vi "User Authentication Schemes Length.vi"(8 "Error In":errorcluster, 10 "Username":string, 11 "Session In":refnum<class "Session.lvclass">) -> (0 "Error Out":errorcluster, 2 "Length":i32, 3 "Sesssion Out":refnum<class "Session.lvclass">)   [LabVIEW 2017, in "Toolkit.lvlib" / "Session.lvclass"]
uses:
  Session.lvclass
  Session.lvclass/Session.ctl
  Toolkit.lvlib
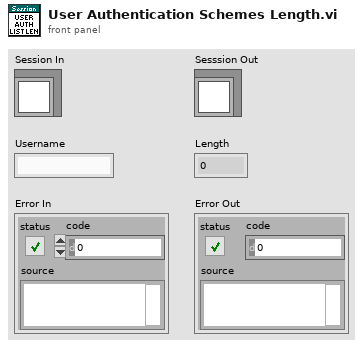
[diagram p1: front panel]
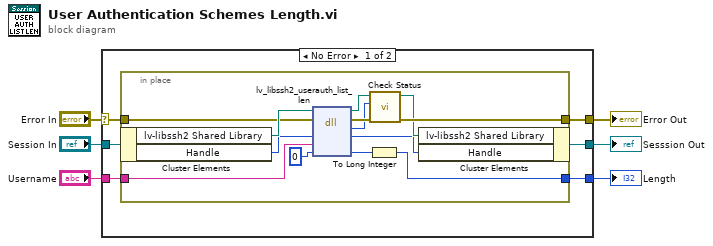
[diagram p0: block diagram]
diagram:
  n1 = case shown="No Error" "Error In" {
    selector: "Error In" -> [w12 w27]
    tunnel: [w9 w27] -> w5
    tunnel: "Session In" -> [w11 w26]
    tunnel: [w10 w26] -> w3
    tunnel: [w8 _] -> w2
    tunnel: "Username" -> [w7 _]
    frame No Error {
      n2 = in-place {
        in-place-border: w12 -> [w21]
        in-place-border: [w20] -> w9
        in-place-border: [w18] -> w8
        in-place-border: w7 -> [w15]
        n3 = in-place-cluster #1(w11) -> ("lv-libssh2 Shared Library"=w25:path, "Handle"=w14:u64)
        n4 = dll-call lib="D:/Users/cfield/Code/Field R&D Services/SSH/LV-LIBSSH2/LabVIEW/trunk/src/Toolkit/Support/lv-libssh2.dll" fn="lv_libssh2_userauth_list_len"(path in=w25, error in=w21, "session"=w14, "username"=w15, "length"=u64 0) -> (path out=w23:path, error out=w24:errorcluster, "result"=w22:i32, "session"=w13:u64, "length"=w16:u64)  [unwired: 2 in]
        n5 = To Long Integer(number=w16) -> (32bit integer=w18:i32)
        n6 = call "Check Status.vi"("Error In"=w24, "Status"=w22, "lv-libssh2 Shared Library In"=w23) -> ("Error Out"=w20:errorcluster, "lv-libssh2 Shared Library Out"=w19:path)  [unwired: 7 in]
        n7 = in-place-cluster #1("lv-libssh2 Shared Library"=w19, "Handle"=w13) -> (w10:refnum<class "Session.lvclass">)
      }
    }
    frame Error {
    }
  }
  "Sesssion Out" <- w3
  "Error Out" <- w5
  "Length" <- w2
